vi "Test.vi"() -> ()   [LabVIEW 2023]
uses:
  <vilib>/Analysis/2dsp.llb/1D Cross Correlation (DBL).vi
  <vilib>/measure/NI_MABase.lvlib
  <vilib>/Analysis/NI_AALPro.lvlib
panel:
  out "x/y":dbl
  out "x*y":dbl
  in  "sampling info":cluster{"Fs":dbl, "#s":dbl}={"Fs"=20000.0, "#s"=10.0}
  out "최대 인덱스 2":i32
  out "최대 인덱스":i32
  out "웨이브폼 그래프 4":waveform(dbl)(graph)
  out "웨이브폼 그래프 3":waveform(dbl)(graph)
  out "웨이브폼 그래프 2":waveform(dbl)(graph)
  out "웨이브폼 그래프":waveform(dbl)(graph)
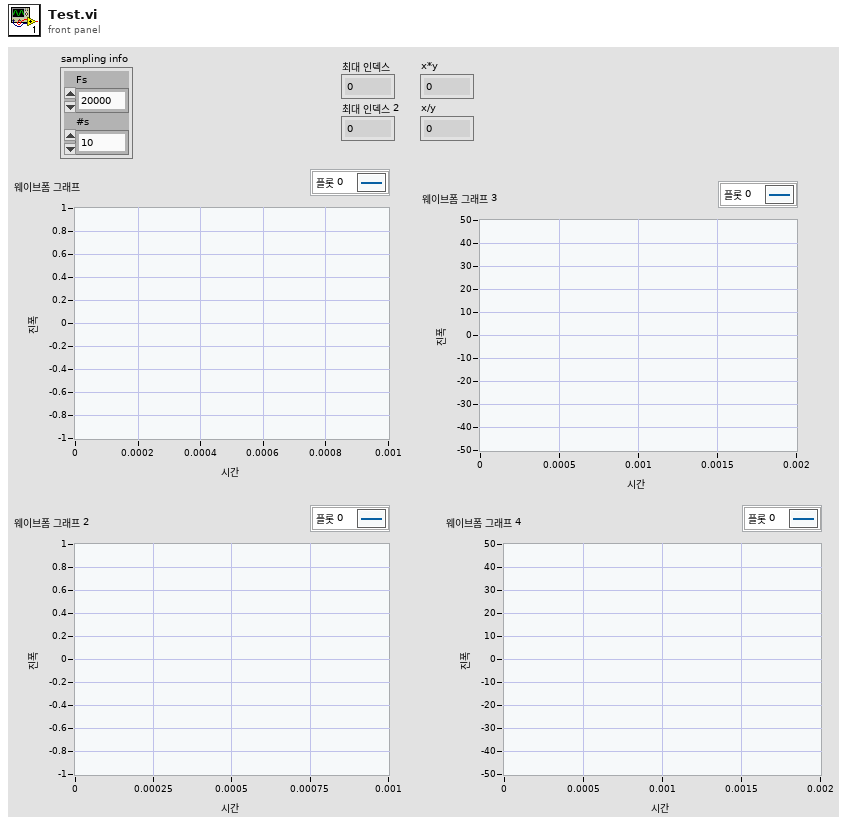
[diagram p1: front panel]
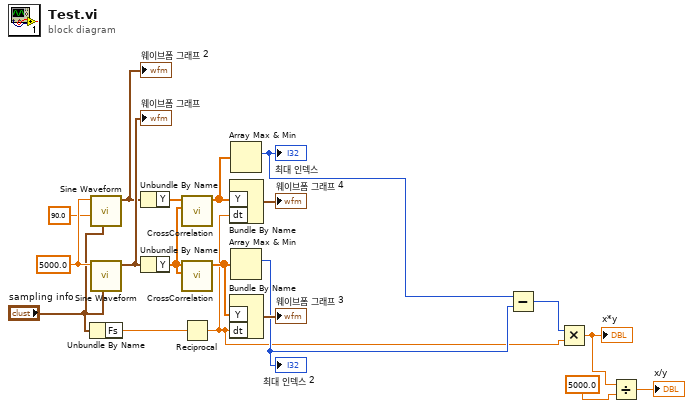
[diagram p0: block diagram]
diagram:
  w19 = 5000.0 ("frequency")
  n1 = Unbundle By Name("sampling info") -> ("Fs"=w12:dbl)
  n2 = call <vilib>:"Sine Waveform.vi"("sampling info"="sampling info", "phase"=90.0, "frequency"=w19) -> ("signal out"=w16:waveform(dbl))  [unwired: 7 in, 1 out]
  "웨이브폼 그래프 2" <- w16
  n3 = call <vilib>:"Sine Waveform.vi"("sampling info"="sampling info", "frequency"=w19) -> ("signal out"=w17:waveform(dbl))  [unwired: 8 in, 1 out]
  "웨이브폼 그래프" <- w17
  n4 = Unbundle By Name(w16) -> ("Y"=w15:dbl[])
  n5 = Unbundle By Name(w17) -> ("Y"=w14:dbl[])
  n6 = call-poly <vilib>:"CrossCorrelation.vi"("Y"=w14, "X"=w15) -> ("Rxy"=w9:dbl[])  [unwired: 8 in, 1 out]
  n7 = call-poly <vilib>:"CrossCorrelation.vi"("Y"=w14, "X"=w14) -> ("Rxy"=w8:dbl[])  [unwired: 8 in, 1 out]
  n8 = Reciprocal(x=w12) -> (1/x=w4:dbl)
  n9 = Bundle By Name("Y"=w9, "dt"=w4) -> (→"웨이브폼 그래프 4":waveform(dbl))  [unwired: 1 in]
  n10 = Bundle By Name("Y"=w8, "dt"=w4) -> (→"웨이브폼 그래프 3":waveform(dbl))  [unwired: 1 in]
  n11 = Array Max & Min(array=w9) -> (max index (indices)=w7:i32)  [unwired: 3 out]
  "최대 인덱스" <- w7
  n12 = Array Max & Min(array=w8) -> (max index (indices)=w6:i32)  [unwired: 3 out]
  "최대 인덱스 2" <- w6
  n13 = Subtract(x=w7, y=w6) -> (x-y=w5:i32)
  n14 = Multiply(x=w5, y=w4) -> (x*y=w2:dbl)
  "x*y" <- w2
  n15 = Divide(x=w2, y=5000.0 ("x")) -> (x/y=→"x/y":dbl)
